vi "46.vi"(1 "逆运动学输入":dbl[](array[numeric])=[0.2, 0.0, 0.3], 2 "1235":dbl[](array[numeric]), 3 "机械臂末端姿态":dbl[][](array[numeric])) -> (0 "逆运动学输出":dbl[](array[numeric])=[0.0, 90.0, 0.0, 0.0, -90.0, -0.0] format="%#.3f")   [LabVIEW 2014]
uses:
  <vilib>/Utility/file.llb/Read From Spreadsheet File (DBL).vi
panel:
  out "angle42":dbl
  out "角度/弧度":dbl
  out "弧度/角度":dbl
  out "az":dbl=1.0
  out "ay":dbl
  out "ax":dbl
  out "angle6":dbl
  out "angle5":dbl
  out "angle4":dbl
  out "angle3":dbl
  out "angle2":dbl
  out "angle1":dbl
  in  "机械臂臂长":dbl[](array[numeric])=[558.0, 764.0, 993.0, 420.0]
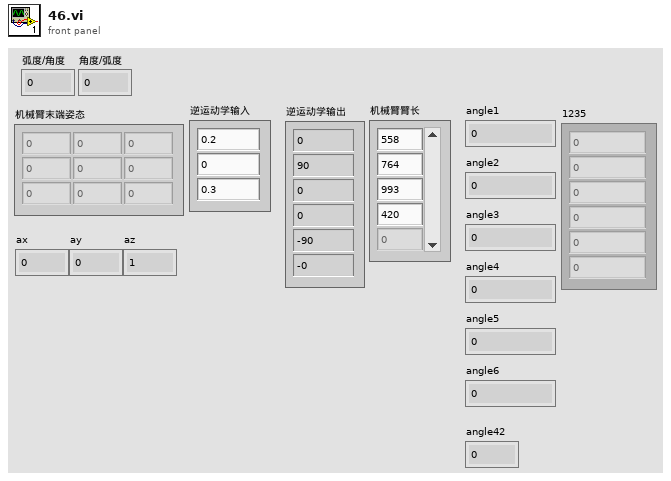
[diagram p1: front panel]
types:
  T1 = typedef "Real Matrix NI_Silver.ctl" = dbl[][]
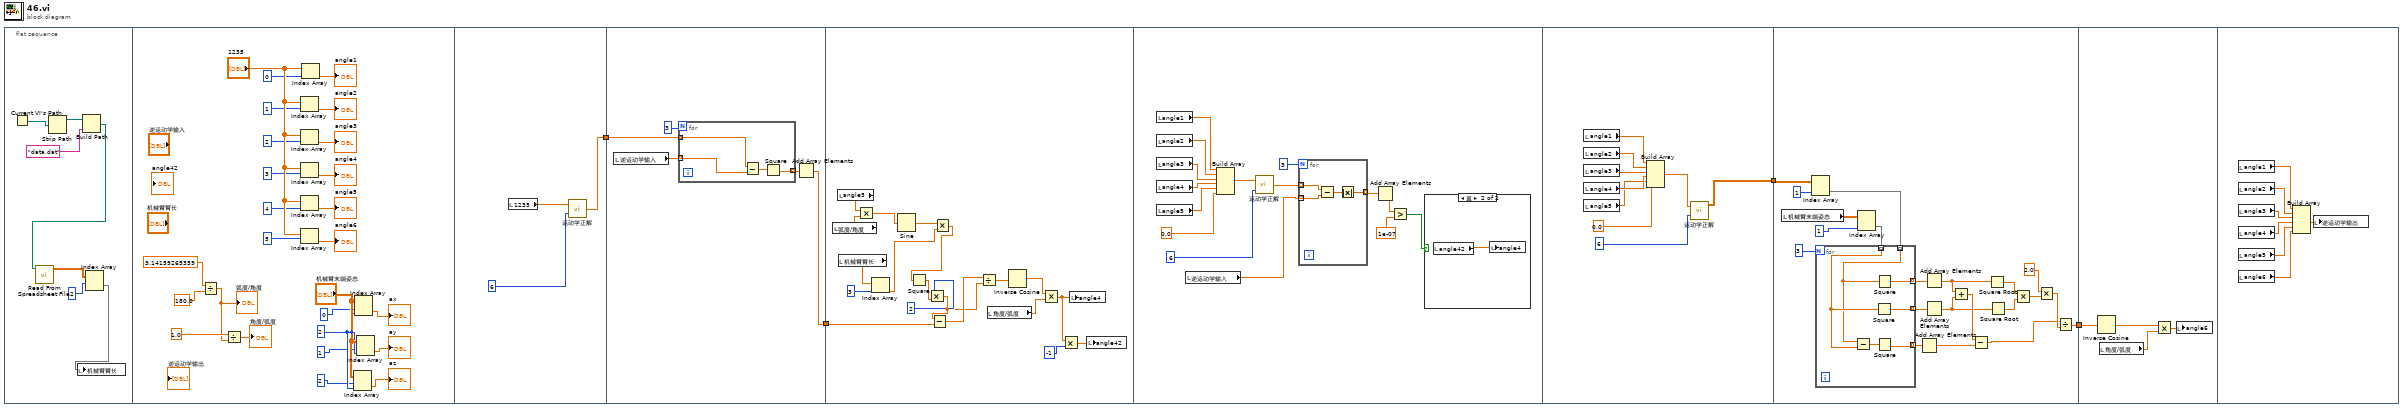
[diagram p0: block diagram]
diagram:
  n1 = flat-sequence {
    tunnel: [w40] -> w4
    tunnel: w4 -> [w43]
    tunnel: [w41] -> w3
    tunnel: w3 -> [w66]
    tunnel: [w89] -> w1
    tunnel: w1 -> [w117]
    tunnel: [w98] -> w2
    tunnel: w2 -> [w128]
    frame #0 {
      n2 = Current VI's Path() -> (path=w8:path)
      n3 = Strip Path(path=w8) -> (stripped path=w7:path)  [unwired: 1 out]
      n4 = Build Path(base path=w7, name or relative path="data.dat") -> (appended path=w5:path)
      n5 = call-poly <vilib>:"Read From Spreadsheet File.vi"("file path (dialog if empty)"=w5) -> ("all rows"=w11:dbl[][])  [unwired: 6 in, 4 out]
      n6 = Index Array(array=w11, index (row)=2) -> (element=w10:dbl[])  [unwired: 1 in]
      n7 = local write "机械臂臂长"(w10) -> ()
    }
    frame #1 {
      w34 = 2
      n8 = Divide(x=3.14159265359, y=180.0) -> (x/y=w26:dbl)
      "弧度/角度" <- w26
      n9 = Divide(x=1.0, y=w26) -> (x/y=→"角度/弧度":dbl)
      n10 = Index Array(array="1235", index=1) -> (element=→"angle2":dbl)
      n11 = Index Array(array="1235", index=2) -> (element=→"angle3":dbl)
      n12 = Index Array(array="1235", index=3) -> (element=→"angle4":dbl)
      n13 = Index Array(array="1235", index=4) -> (element=→"angle5":dbl)
      n14 = Index Array(array="1235", index=5) -> (element=→"angle6":dbl)
      n15 = Index Array(array="1235", index=0) -> (element=→"angle1":dbl)
      n16 = Index Array(array="机械臂末端姿态", index (row)=2, index (col)=w34) -> (element=→"az":dbl)
      n17 = Index Array(array="机械臂末端姿态", index (row)=0, index (col)=w34) -> (element=→"ax":dbl)
      n18 = Index Array(array="机械臂末端姿态", index (row)=1, index (col)=w34) -> (element=→"ay":dbl)
    }
    frame #2 {
      n19 = local read "1235"() -> (w38:dbl[])
      n20 = call "运动学正解.vi"("正运动学输入"=w38, "关节数"=6) -> ("正解输出"=w40:dbl[])  [unwired: 2 out]
    }
    frame #3 {
      n21 = local read "逆运动学输入"() -> (w42:dbl[])
      n22 = for {
        N: 3 -> [_]
        tunnel: [w48] -> w44 mode=indexing
        tunnel: w43 -> [w47] mode=indexing
        tunnel: w42 -> [w46] mode=indexing
        n23 = Subtract(x=w47, y=w46) -> (x-y=w49:dbl)
        n24 = Square(x=w49) -> (x^2=w48:dbl)
      }
      n25 = Add Array Elements(numeric array=w44) -> (sum=w41:dbl)
    }
    frame #4 {
      n26 = local read "弧度/角度"() -> (w60:dbl)
      n27 = local read "angle5"() -> (w61:dbl)
      n28 = local read "机械臂臂长"() -> (w68:dbl[])
      n29 = Multiply(x=w61, y=w60) -> (x*y=w59:dbl)
      n30 = Index Array(array=w68, index=3) -> (element=w64:dbl)
      n31 = Sine(x=w59) -> (sin(x)=w65:dbl)
      n32 = Multiply(x=w65, y=w64) -> (x*y=w56:dbl)
      n33 = Square(x=w56) -> (x^2=w55:dbl)
      n34 = Multiply(x=2, y=w55) -> (x*y=w53:dbl)
      n35 = Subtract(x=w53, y=w66) -> (x-y=w63:dbl)
      n36 = Divide(x=w63, y=w53) -> (x/y=w62:dbl)
      n37 = local read "角度/弧度"() -> (w58:dbl)
      n38 = Inverse Cosine(1:w62) -> (0:w57:dbl)
      n39 = Multiply(x=w57, y=w58) -> (x*y=w51:dbl)
      n40 = Multiply(x=w51, y=-1) -> (x*y=w50:dbl)
      n41 = local write "angle4"(w51) -> ()
      n42 = local write "angle42"(w50) -> ()
    }
    frame #5 {
      n43 = local read "angle1"() -> (w83:dbl)
      n44 = local read "angle2"() -> (w82:dbl)
      n45 = local read "angle3"() -> (w81:dbl)
      n46 = local read "angle4"() -> (w80:dbl)
      n47 = local read "angle5"() -> (w79:dbl)
      n48 = local read "逆运动学输入"() -> (w73:dbl[])
      n49 = Build Array(w83, w82, w81, w80, w79, 0.0) -> (w77:dbl[])
      n50 = call "运动学正解.vi"("正运动学输入"=w77, "关节数"=6) -> ("正解输出"=w74:dbl[])  [unwired: 2 out]
      n51 = for {
        N: 3 -> [_]
        tunnel: w74 -> [w88] mode=indexing
        tunnel: w73 -> [w87] mode=indexing
        tunnel: [w85] -> w72 mode=indexing
        n52 = Subtract(x=w88, y=w87) -> (x-y=w86:dbl)
        n53 = Absolute Value(x=w86) -> (abs(x)=w85:dbl)
      }
      n54 = Add Array Elements(numeric array=w72) -> (sum=w71:dbl)
      n55 = Greater?(x=w71, y=1e-07) -> (0:w69:bool)
      n56 = case shown="真" w69 {
        frame False {
        }
        frame True {
          n57 = local read "angle42"() -> (w84:dbl)
          n58 = local write "angle4"(w84) -> ()
        }
      }
    }
    frame #6 {
      n59 = local read "angle1"() -> (w97:dbl)
      n60 = local read "angle2"() -> (w96:dbl)
      n61 = local read "angle3"() -> (w95:dbl)
      n62 = local read "angle4"() -> (w94:dbl)
      n63 = local read "angle5"() -> (w93:dbl)
      n64 = Build Array(w97, w96, w95, w94, w93, 0.0) -> (w91:dbl[])
      n65 = call "运动学正解.vi"("正运动学输入"=w91, "关节数"=6) -> ("Tx"=w89:T1)  [unwired: 2 out]
    }
    frame #7 {
      n66 = local read "机械臂末端姿态"() -> (w115:dbl[][])
      n67 = Index Array(array=w117, index (col)=1) -> (element=w113:dbl[])  [unwired: 1 in]
      n68 = Index Array(array=w115, index (col)=1) -> (element=w112:dbl[])  [unwired: 1 in]
      n69 = for {
        N: 3 -> [_]
        tunnel: w113 -> [w121] mode=indexing
        tunnel: w112 -> [w122] mode=indexing
        tunnel: [w123] -> w111 mode=indexing
        tunnel: [w120] -> w110 mode=indexing
        tunnel: [w119] -> w109 mode=indexing
        n70 = Subtract(x=w121, y=w122) -> (x-y=w124:dbl)
        n71 = Square(x=w122) -> (x^2=w119:dbl)
        n72 = Square(x=w121) -> (x^2=w120:dbl)
        n73 = Square(x=w124) -> (x^2=w123:dbl)
      }
      n74 = Add Array Elements(numeric array=w111) -> (sum=w107:dbl)
      n75 = Add Array Elements(numeric array=w110) -> (sum=w106:dbl)
      n76 = Add Array Elements(numeric array=w109) -> (sum=w105:dbl)
      n77 = Add(x=w106, y=w105) -> (x+y=w108:dbl)
      n78 = Subtract(x=w108, y=w107) -> (x-y=w99:dbl)
      n79 = Square Root(x=w106) -> (sqrt(x)=w103:dbl)
      n80 = Square Root(x=w105) -> (sqrt(x)=w104:dbl)
      n81 = Multiply(x=w103, y=w104) -> (x*y=w102:dbl)
      n82 = Multiply(x=2.0, y=w102) -> (x*y=w100:dbl)
      n83 = Divide(x=w99, y=w100) -> (x/y=w98:dbl)
    }
    frame #8 {
      n84 = Inverse Cosine(1:w128) -> (0:w126:dbl)
      n85 = local read "角度/弧度"() -> (w127:dbl)
      n86 = Multiply(x=w126, y=w127) -> (x*y=w125:dbl)
      n87 = local write "angle6"(w125) -> ()
    }
    frame #9 {
      n88 = local read "angle1"() -> (w135:dbl)
      n89 = local read "angle2"() -> (w134:dbl)
      n90 = local read "angle3"() -> (w133:dbl)
      n91 = local read "angle4"() -> (w132:dbl)
      n92 = local read "angle5"() -> (w131:dbl)
      n93 = local read "angle6"() -> (w130:dbl)
      n94 = Build Array(w135, w134, w133, w132, w131, w130) -> (w129:dbl[])
      n95 = local write "逆运动学输出"(w129) -> ()
    }
  }
